vi "Extract axis properties.vi"(0 "Name":T2=enum."AxisX", 1 "All servo status":T1[](array[typedef]) {"Last update" format="%<%H:%M:%S>T"}) -> (7 "Servo":T1 {"Last update" format="%<%H:%M:%S>T"}, 8 "Index":i32, 9 "Found?":bool)   [LabVIEW 2021]
uses:
  Subsystem modules/Servo drive module/ctl/Axis names.ctl
  Datatypes/Single servo status.ctl
  Subsystem modules/Servo drive module/Servo drive module.lvlib
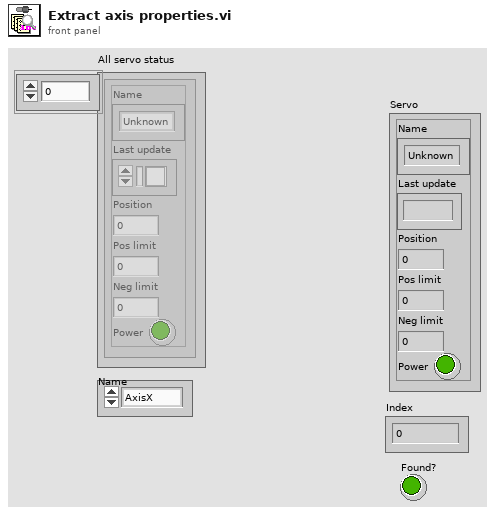
[diagram p1: front panel]
types:
  T1 = typedef "Single servo status.ctl" = cluster{"Name":T2, "Last update":timestamp, "Position":dbl, "Pos limit":dbl, "Neg limit":dbl, "Power":bool}
  T2 = typedef "Servo drive module.lvlib/Axis names.ctl" = enum16{"Unknown", "AxisX", "AxisY", "AxisZ_left", "AxisZ_middle", "AxisZ_right"}
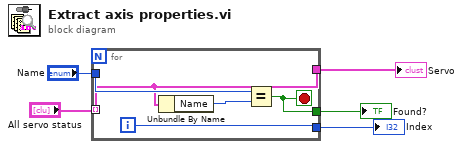
[diagram p0: block diagram]
diagram:
  n1 = for {
    tunnel: "All servo status" -> [w7] mode=indexing
    tunnel: "Name" -> [w9]
    tunnel: [w8] -> w4
    tunnel: [w7] -> w1
    tunnel: [w6] -> w3
    i -> [w8]
    stop <- w6 stop-if-true
    n2 = Unbundle By Name(w7) -> ("Name"=w10:T2)
    n3 = Equal?(x=w9, y=w10) -> (x = y?=w6:bool)
  }
  "Index" <- w4
  "Found?" <- w3
  "Servo" <- w1
